vi "No Heartbeat.vi"(8 "error in (no error)":errorcluster, 10 "No Heartbeat?":bool) -> (0 "error out":errorcluster)   [LabVIEW 2023, in "Error Handling.lvlib"]
doc: "Send Error VI to No Initial Heart State, causing this to send all queues to normal mode"
uses:
  Error Handling.lvlib
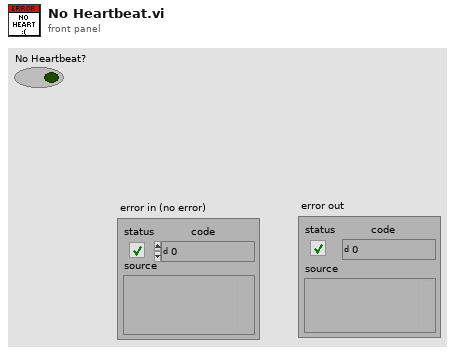
[diagram p1: front panel]
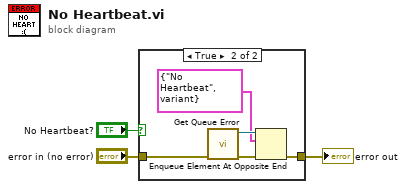
[diagram p0: block diagram]
diagram:
  n1 = case shown="True" "No Heartbeat?" {
    tunnel: "error in (no error)" -> [w4 w6]
    tunnel: [w4 w5] -> w1
    frame False {
    }
    frame True {
      n2 = call "Get Queue Error.vi"("error in (no error)"=w6) -> ("error out"=w8:errorcluster, "Error Queue"=w9:refnum<queue>)  [unwired: 8 in, 1 out]
      n3 = Enqueue Element At Opposite End(queue=w9, element=cluster{string, variant} {"No Heartbeat", variant}, error in (no error)=w8) -> (error out=w5:errorcluster)  [unwired: 1 in, 2 out]
    }
  }
  "error out" <- w1
